vi "AuxEC_CAL 2016.vi"(6 "Sensor Cluster":T1, 7 "Array in":refnum<k24>[](array[refnum]), 8 "error in (no error)":errorcluster, 9 "Descriptions":string[](array[string]), 11 "Aux Sensor":i32=3) -> (0 "error out":errorcluster, 2 "Aux Sensor\nHigh Value":dbl format="%.4f", 3 "Aux Sensor\nLow Value":dbl format="%.4f", 4 "Sensor Cluster 2":T1, 5 "Array out":refnum<k24>[](array[refnum]))   [LabVIEW 2016]
uses:
  C:/Cascade-lv16-64/builds/Waterloo Main Program/cascade/data/ULx_LV.dll
  builds/Waterloo Main Program/cascade/data/ULx_LV.dll
  controls/MCC DAQ Readings.ctl
panel:
  out "Aux Sensor\nVoltage 2 (V)":dbl format="%.4f"
  out "delta Parameter":dbl
  out "Aux Sensor\nVoltage 1 (V)":dbl format="%.4f"
  in  "stop":bool
  in  "start":bool
  # "AUX3/EC SENSOR CALIBRATION"
  # "Connect Low Level Sample.\n Press start."
  # "Connect High Level Sample.  Press stop"
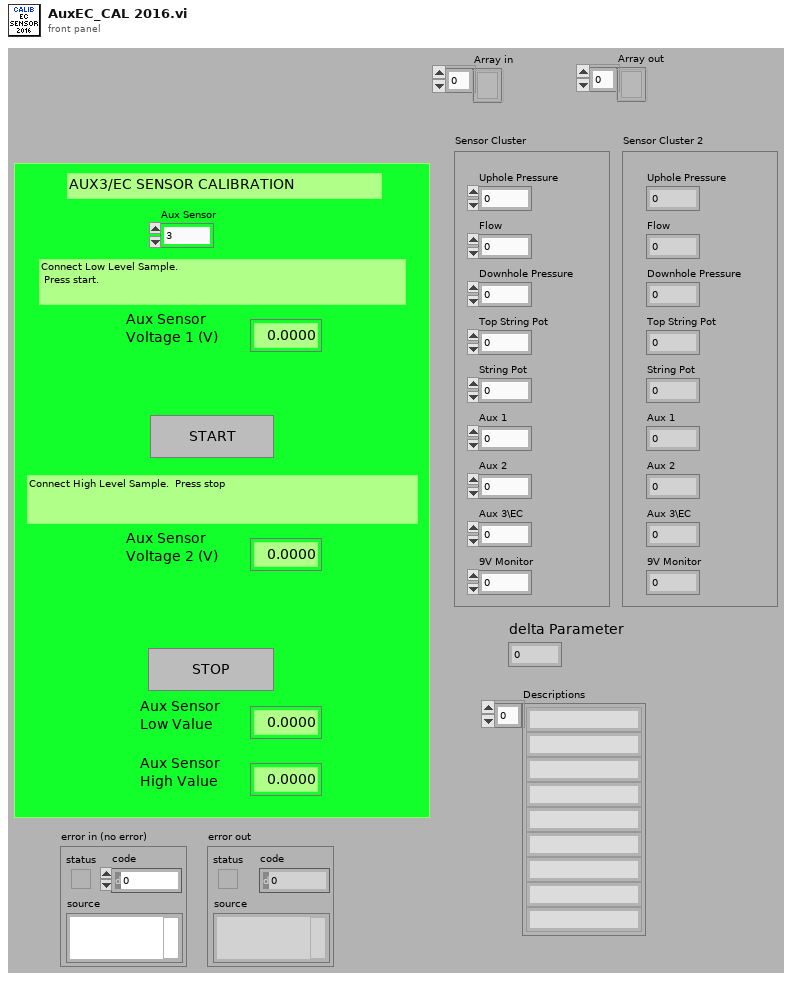
[diagram p1: front panel]
types:
  T1 = typedef "MCC DAQ Readings.ctl" = cluster{"Uphole Pressure":dbl, "Flow":dbl, "Downhole Pressure":dbl, "Top String Pot":dbl, "String Pot":dbl, "Aux 1":dbl, "Aux 2":dbl, "Aux 3\\EC":dbl, "9V Monitor":dbl}
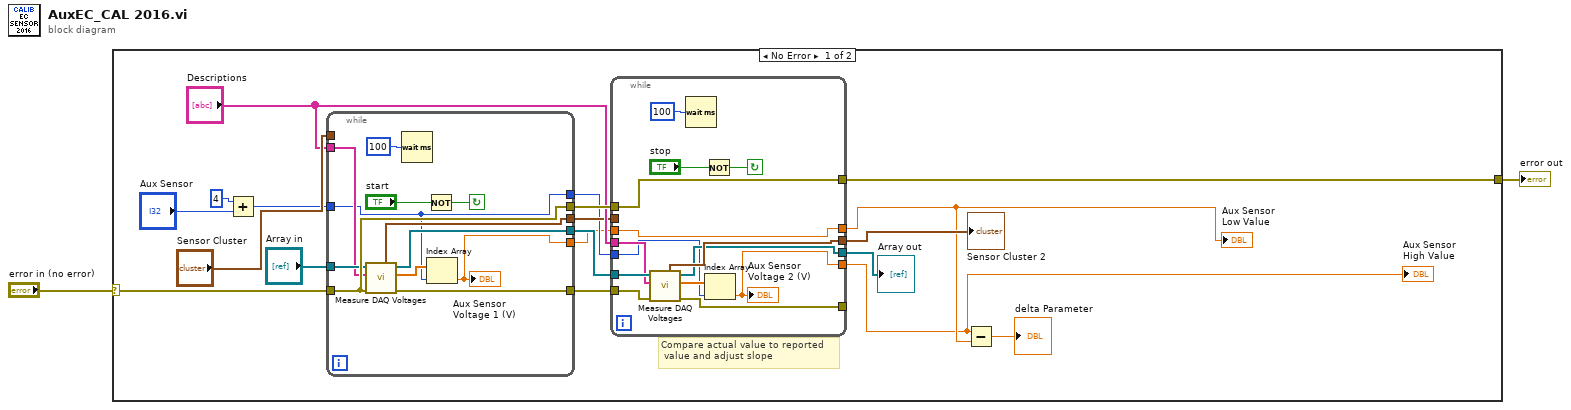
[diagram p0: block diagram]
diagram:
  n1 = case shown="No Error" "error in (no error)" {
    selector: "error in (no error)" -> [w21 w48]
    tunnel: [w19 w48] -> w2
    frame No Error {
      # "Compare actual value to reported\n value and adjust slope"
      n2 = Add(x=4, y="Aux Sensor") -> (x+y=w7:i32)
      n3 = while {
        tunnel: [w30] -> w20
        tunnel: w21 -> [w30]
        tunnel: "Array in" -> [w29]
        tunnel: "Sensor Cluster" -> [_]
        tunnel: "Descriptions" -> [w26]
        tunnel: [w27] -> w13
        tunnel: [w28] -> w15
        tunnel: w7 -> [w23]
        tunnel: [w25] -> w10
        tunnel: [w23] -> w6
        tunnel: [w22] -> w5
        stop <- w32 continue-if-true
        n4 = call "Measure DAQ Voltages.vi"("error in (no error)"=w30, "Descriptions"=w26, "Array in"=w29) -> ("error in (no error) 2"=w25:errorcluster, "Raw Voltages"=w24:dbl[], "Array out"=w28:refnum<k24>[], "Sensor Cluster"=w27:T1)  [unwired: 5 in]
        n5 = Wait (ms)(milliseconds to wait=u32 100) -> ()  [unwired: 1 out]
        n6 = Not(x="start") -> (.not. x?=w32:bool)
        n7 = Index Array(array=w24, index=w23) -> (element=w22:dbl)
        "Aux Sensor\nVoltage 1 (V)" <- w22
      }
      n8 = while {
        tunnel: [w34] -> w4
        tunnel: [w35] -> w3
        tunnel: w20 -> [w45]
        tunnel: [w45] -> w19
        tunnel: "Descriptions" -> [w38]
        tunnel: w15 -> [w39]
        tunnel: [w40] -> w14
        tunnel: w13 -> [_]
        tunnel: [w41] -> w12
        tunnel: w10 -> [w43]
        tunnel: [w42] -> _
        tunnel: w6 -> [w36]
        tunnel: w5 -> [w34]
        stop <- w47 continue-if-true
        n9 = call "Measure DAQ Voltages.vi"("error in (no error)"=w43, "Descriptions"=w38, "Array in"=w39) -> ("error in (no error) 2"=w42:errorcluster, "Raw Voltages"=w37:dbl[], "Array out"=w40:refnum<k24>[], "Sensor Cluster"=w41:T1)  [unwired: 5 in]
        n10 = Wait (ms)(milliseconds to wait=u32 100) -> ()  [unwired: 1 out]
        n11 = Not(x="stop") -> (.not. x?=w47:bool)
        n12 = Index Array(array=w37, index=w36) -> (element=w35:dbl)
        "Aux Sensor\nVoltage 2 (V)" <- w35
      }
      "Sensor Cluster 2" <- w12
      "Array out" <- w14
      "Aux Sensor\nLow Value" <- w4
      "Aux Sensor\nHigh Value" <- w3
      n13 = Subtract(x=w3, y=w4) -> (x-y=→"delta Parameter":dbl)
    }
    frame Error {
    }
  }
  "error out" <- w2
